vi "排气扇运行流程.vi"   [LabVIEW 2016, in "采配水.lvlib"]
uses:
  <vilib>/ptbypt/NI_PtbyPt.lvlib
types:
  T1 = cluster{"功能开关":enum16{"关闭", "开启"}, "排气扇开启温度":dbl, "排气扇关闭温度":dbl}
  T2 = cluster{"蓄电池电压":dbl, "室温":dbl, "湿度":dbl, "水浸报警":bool, "烟雾报警":bool, "门禁1状态":bool, "门禁2状态":bool}
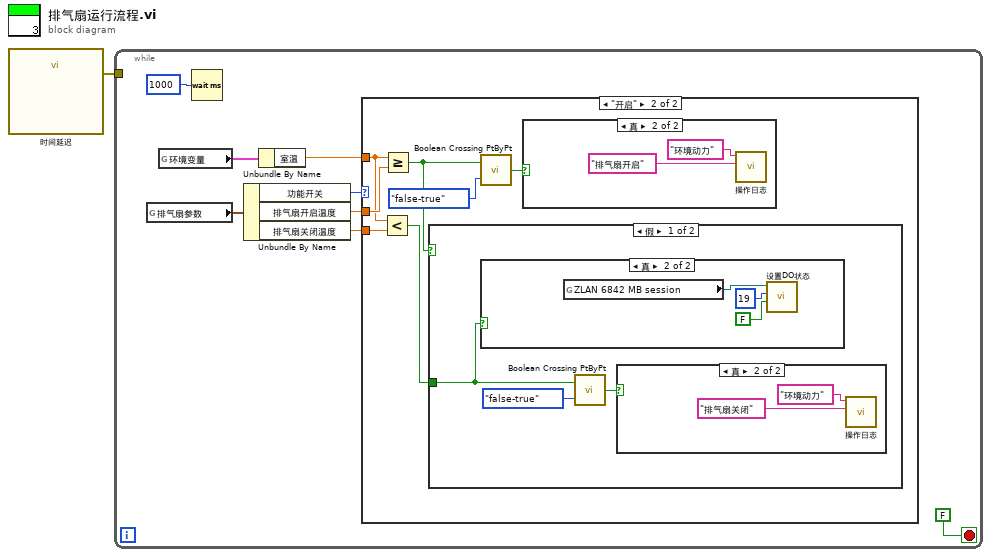
[diagram p0: block diagram]
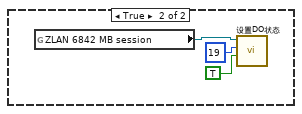
[diagram p6: hidden frame]
diagram:
  n1 = call "时间延迟"() -> ("error out"=w1:errorcluster)  [unwired: 11 in]
  n2 = while {
    tunnel: w1 -> [_]
    stop <- FALSE stop-if-true
    n3 = global read "通讯全局变量断电保存.vi" "排气扇参数"() -> (w9:T1)
    n4 = global read "通讯全局变量.vi" "环境变量"() -> (w3:T2)
    n5 = Wait (ms)(milliseconds to wait=u32 1000 ("等待时间（毫秒）")) -> ()  [unwired: 1 out]
    n6 = Unbundle By Name(w9) -> ("功能开关"=w8:enum16{"关闭", "开启"}, "排气扇开启温度"=w7:dbl, "排气扇关闭温度"=w6:dbl)
    n7 = Unbundle By Name(w3) -> ("室温"=w2:dbl)
    n8 = case shown="\"开启\"" w8 {
      tunnel: w7 -> [_ w12]
      tunnel: w6 -> [_ w11]
      tunnel: w2 -> [_ w10]
      frame "关闭", Default {
      }
      frame "开启" {
        n9 = Less?(x=w10, y=w11) -> (x < y?=w16:bool)
        n10 = Greater Or Equal?(x=w10, y=w12) -> (x >= y?=w15:bool)
        n11 = case shown="假" w15 {
          tunnel: w16 -> [w19 _]
          frame False {
            n12 = case shown="真" w19 {
              frame False {
              }
              frame True {
                n13 = global read "通讯全局变量.vi" "ZLAN 6842 MB session"() -> (w26:refnum<class "MB_Master.lvclass">)
                n14 = call "设置DO状态.vi"("value"=FALSE, "address"=u16 19, "MB session in"=w26) -> ()  [unwired: 7 in, 2 out]
              }
            }
            n15 = call <vilib>:"Boolean Crossing PtByPt.vi"("direction"=enum16{"either", "false-true", "true-false"}."false-true", "input"=w19) -> ("crossing"=w20:bool)  [unwired: 1 in]
            n16 = case shown="真" w20 {
              frame False {
              }
              frame True {
                n17 = call "操作日志.vi"("日志信息"="排气扇关闭", "设备"="环境动力") -> ()  [unwired: 9 in, 1 out]
              }
            }
          }
          frame True {
            n18 = global read "通讯全局变量.vi" "ZLAN 6842 MB session"() -> (w29:refnum<class "MB_Master.lvclass">)
            n19 = call "设置DO状态.vi"("value"=TRUE, "address"=u16 19, "MB session in"=w29) -> ()  [unwired: 7 in, 2 out]
          }
        }
        n20 = call <vilib>:"Boolean Crossing PtByPt.vi"("direction"=enum16{"either", "false-true", "true-false"}."false-true", "input"=w15) -> ("crossing"=w14:bool)  [unwired: 1 in]
        n21 = case shown="真" w14 {
          frame False {
          }
          frame True {
            n22 = call "操作日志.vi"("日志信息"="排气扇开启", "设备"="环境动力") -> ()  [unwired: 9 in, 1 out]
          }
        }
      }
    }
  }
